vi "Compute DistanceTo AprilTag Ver 3.vi"(6 "Robot Calibration Cluster":T1={"Camera Height on robot (in)"=6.0, "Camera Angle on the robot (deg)"=5.0, "Camera FOV Top to Bottom View Angle (deg)"=52.3, "Camera FOV Left to Right View Angle (deg)"=92.0, "Target size (in)"=6.5, "Distance to front of bumper (in)"=0.0, "Focal Length (mm)"=10.0, "Yaw Slope"=9.75, "Yaw Offset"=10.0} {"Yaw Offset" format="%#_13g"; "Yaw Slope" format="%#_13g"; "Camera FOV Left to Right View Angle (deg)" format="%#_13g"; "Focal Length (mm)" format="%#_13g"; "Distance to front of bumper (in)" format="%#_13g"; "Target size (in)" format="%#_13g"; "Camera FOV Top to Bottom View Angle (deg)" format="%#_13g"; "Camera Angle on the robot (deg)" format="%#_13g"; "Camera Height on robot (in)" format="%#_13g"}, 8 "Height to center of target from floor (hp (in))":dbl=10.875 format="%#_13g", 9 "Screen resolution pixels Height (Ry)":dbl=600.0 format="%#_13g", 10 "Target Vertical pixels bottom - top (pixels)":dbl=-46.076202392578125 format="%#_13g") -> (2 "Distance from target to camera (in) 2":dbl format="%.2f", 3 "Distance from target to bumper (in)":dbl format="%.2f")   [LabVIEW 2023]
uses:
  Camera Info.ctl
panel:
  out "sqrt(x)":dbl
  # "These Items are inputs"
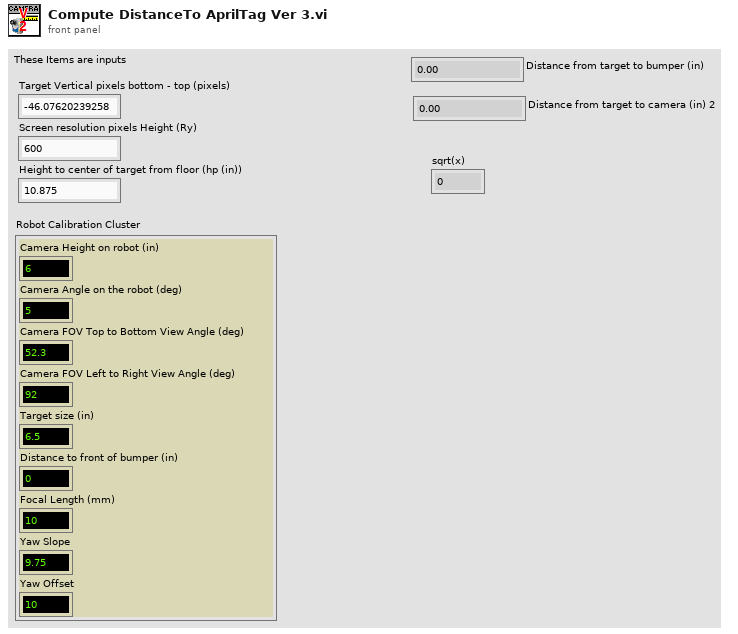
[diagram p1: front panel]
types:
  T1 = typedef "Camera Info.ctl" = cluster{"Camera Height on robot (in)":dbl, "Camera Angle on the robot (deg)":dbl, "Camera FOV Top to Bottom View Angle (deg)":dbl, "Camera FOV Left to Right View Angle (deg)":dbl, "Target size (in)":dbl, "Distance to front of bumper (in)":dbl, "Focal Length (mm)":dbl, "Yaw Slope":dbl, "Yaw Offset":dbl}
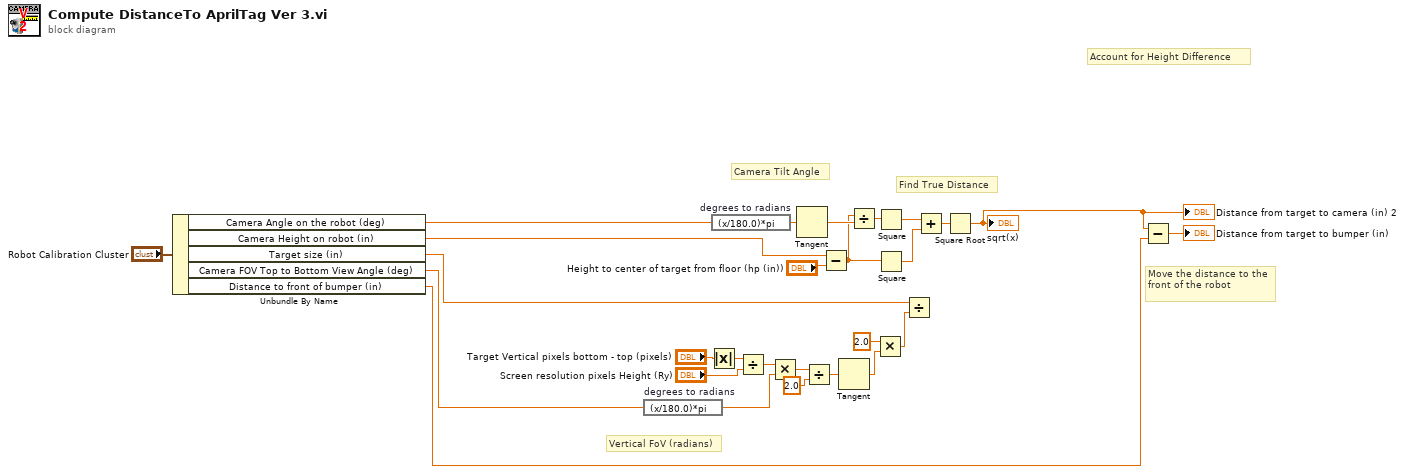
[diagram p0: block diagram]
diagram:
  # "Move the distance to the front of the robot"
  # "Camera Tilt Angle"
  # "Account for Height Difference"
  # "Find True Distance"
  # "Vertical FoV (radians)"
  n1 = Unbundle By Name("Robot Calibration Cluster") -> ("Camera Angle on the robot (deg)"=w9:dbl, "Camera Height on robot (in)"=w26:dbl, "Target size (in)"=w24:dbl, "Camera FOV Top to Bottom View Angle (deg)"=w23:dbl, "Distance to front of bumper (in)"=w21:dbl)
  n2 = expression code="(x/180.0)*pi" "degrees to radians"(w23) -> (w16:dbl)
  n3 = Absolute Value(x="Target Vertical pixels bottom - top (pixels)") -> (abs(x)=w19:dbl)
  n4 = expression code="(x/180.0)*pi" "degrees to radians"(w9) -> (w8:dbl)
  n5 = Divide(x=w19, y="Screen resolution pixels Height (Ry)") -> (x/y=w17:dbl)
  n6 = Multiply(x=w17, y=w16) -> (x*y=w15:dbl)
  n7 = Tangent(1:w8) -> (0:w7:dbl)
  n8 = Divide(x=w15, y=2.0) -> (x/y=w13:dbl)
  n9 = Subtract(x=w26, y="Height to center of target from floor (hp (in))") -> (x-y=w5:dbl)
  n10 = Tangent(1:w13) -> (0:w11:dbl)
  n11 = Divide(x=w5, y=w7) -> (x/y=w6:dbl)
  n12 = Multiply(x=2.0, y=w11) -> (x*y=w10:dbl)
  n13 = Square(x=w6) -> (x^2=w4:dbl)
  n14 = Square(x=w5) -> (x^2=w3:dbl)
  n15 = Divide(x=w24, y=w10) -> ()  [unwired: 1 out]
  n16 = Add(x=w4, y=w3) -> (x+y=w2:dbl)
  n17 = Square Root(x=w2) -> (sqrt(x)=w1:dbl)
  "Distance from target to camera (in) 2" <- w1
  "sqrt(x)" <- w1
  n18 = Subtract(x=w1, y=w21) -> (x-y=→"Distance from target to bumper (in)":dbl)
